vi "DSKGraph.vi"() -> ()   [LabVIEW 2023]
panel:
  out "Waveform Chart":dbl[](graph)
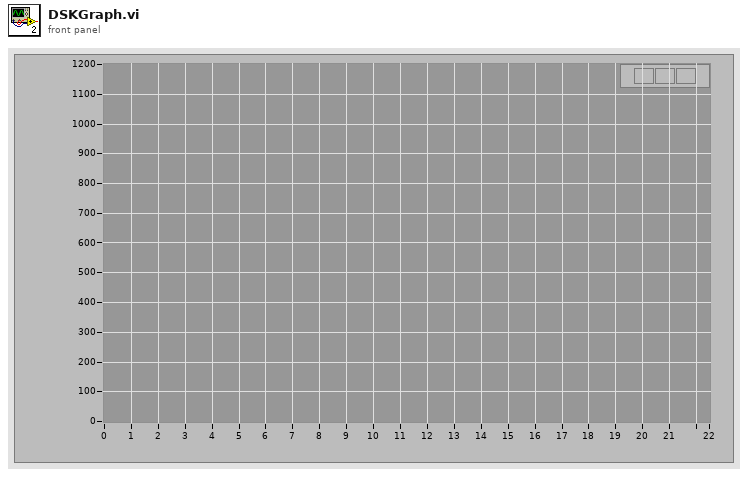
[diagram p1: front panel]
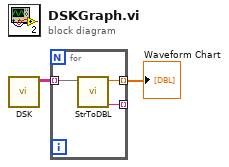
[diagram p0: block diagram]
diagram:
  n1 = call "DSK.vi"() -> ("Current Transaction"=w2:string[][])  [unwired: 8 in, 3 out]
  n2 = for {
    tunnel: w2 -> [w5] mode=indexing
    tunnel: [w4] -> w1 mode=indexing
    tunnel: [w3] -> _ mode=indexing
    n3 = call "StrToDBL.vi"("Array 2"=w5) -> ("Date"=w3:string, "number"=w4:dbl)  [unwired: 9 in]
  }
  "Waveform Chart" <- w1
